vi "Write App Log.vi"(8 "error in (no error)":errorcluster, 10 "String To Write":string, 11 "Path in":refnum<vi>) -> (0 "error out":errorcluster, 2 "Is Valid?":bool)   [LabVIEW 2024]
uses:
  Variables/Download Confrigurations.vi
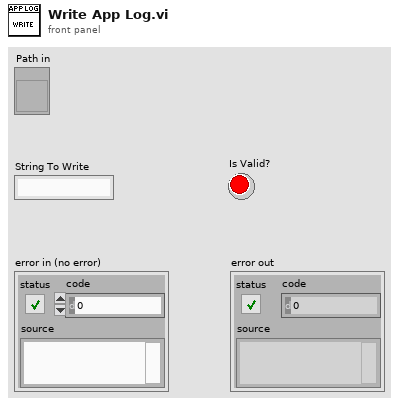
[diagram p1: front panel]
types:
  T1 = enum16{"open", "replace", "create", "open or create", "replace or create", "replace or create with confirmation"}
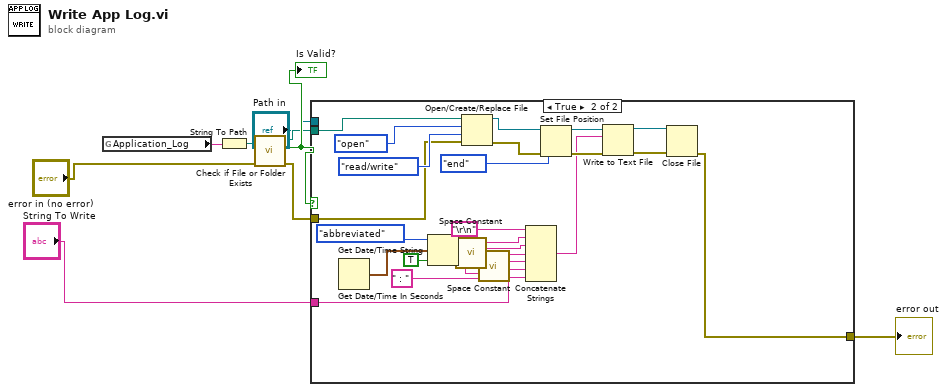
[diagram p0: block diagram]
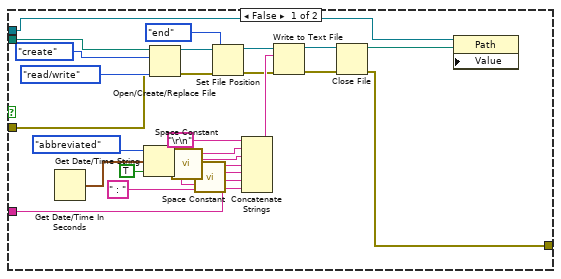
[diagram p2: hidden frame]
diagram:
  n1 = global read "Download Confrigurations.vi" "Application_Log"() -> (w2:string)
  n2 = String To Path(string=w2) -> (path=w3:path)
  n3 = call <vilib>:"Check if File or Folder Exists.vi"("error in (no error)"="error in (no error)", "path"=w3) -> ("error out"=w6:errorcluster, "file or folder exists?"=w9:bool, "dup path"=w5:path)  [unwired: 7 in]
  "Is Valid?" <- w9
  n4 = case shown="True" w9 {
    tunnel: w5 -> [w34 w57]
    tunnel: w6 -> [w31 w54]
    tunnel: "String To Write" -> [w21 w39]
    tunnel: [w11 w35] -> w8
    tunnel: "Path in" -> [w10 _]
    frame False {
      n5 = Get Date/Time In Seconds() -> (seconds since 1Jan1904=w30:timestamp)
      n6 = Get Date/Time String(date format (0)=enum16{"short", "long", "abbreviated"}."abbreviated", seconds (now)=w30, want seconds? (F)=TRUE) -> (date string=w27:string, time string=w25:string)
      n7 = Open/Create/Replace File(file path (use dialog)=w34, error in=w31, operation (0:open)=T1."create", access (0:read/write)=enum16{"read/write", "read-only", "write-only"}."read/write") -> (refnum out=w20:refnum<file>, error out=w18:errorcluster)  [unwired: 2 in, 1 out]
      n8 = call <vilib>:"Space Constant.vi"() -> ("String"=w26:string)
      n9 = call <vilib>:"Space Constant.vi"() -> ("String"=w24:string)
      n10 = Set File Position(refnum=w20, from (0:start)=enum16{"start", "end", "current"}."end", error in=w18) -> (refnum out=w17:refnum<file>, error out=w15:errorcluster)  [unwired: 1 in]
      n11 = Concatenate Strings("\r\n", w27, w26, w25, w24, " : ", w21) -> (w16:string)
      n12 = Write to Text File(file (use dialog)=w17, text=w16, error in=w15) -> (refnum out=w14:refnum<file>, error out=w13:errorcluster)  [unwired: 1 in, 1 out]
      n13 = Close File(refnum=w14, error in=w13) -> (path=w12:path, error out=w11:errorcluster)
      n14 = property class="Path"(reference=w10, "Value"=w12) -> ()  [unwired: 1 in, 2 out]
    }
    frame True {
      n15 = Get Date/Time In Seconds() -> (seconds since 1Jan1904=w48:timestamp)
      n16 = Get Date/Time String(date format (0)=enum16{"short", "long", "abbreviated"}."abbreviated", seconds (now)=w48, want seconds? (F)=TRUE) -> (date string=w45:string, time string=w43:string)
      n17 = call <vilib>:"Space Constant.vi"() -> ("String"=w44:string)
      n18 = Open/Create/Replace File(file path (use dialog)=w57, error in=w54, operation (0:open)=T1."open", access (0:read/write)=enum16{"read/write", "read-only", "write-only"}."read/write") -> (refnum out=w53:refnum<file>, error out=w51:errorcluster)  [unwired: 2 in, 1 out]
      n19 = call <vilib>:"Space Constant.vi"() -> ("String"=w42:string)
      n20 = Concatenate Strings("\r\n", w45, w44, w43, w42, " : ", w39) -> (w38:string)
      n21 = Set File Position(refnum=w53, from (0:start)=enum16{"start", "end", "current"}."end", error in=w51) -> (refnum out=w50:refnum<file>, error out=w49:errorcluster)  [unwired: 1 in]
      n22 = Write to Text File(file (use dialog)=w50, text=w38, error in=w49) -> (refnum out=w37:refnum<file>, error out=w36:errorcluster)  [unwired: 1 in, 1 out]
      n23 = Close File(refnum=w37, error in=w36) -> (error out=w35:errorcluster)  [unwired: 1 out]
    }
  }
  "error out" <- w8
